vi "LWXPS_OptionalModuleExecute.vi"(6 "LabVIEW error IN":errorcluster, 8 "Module File Name":string, 9 "XPS Reference IN":refnum<k24>) -> (0 "LabVIEW error OUT":errorcluster, 1 "XPS Error String":string, 2 "Returned error code":i32, 3 "XPS Reference OUT":refnum<k24>)   [LabVIEW 2014]
uses:
  D:/XPSQ8_LabView_Library/Development/Source/Dll/Newport.XPS.CommandInterface.dll
  Dll/Newport.XPS.CommandInterface.dll
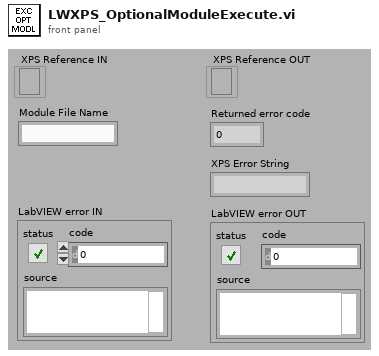
[diagram p1: front panel]
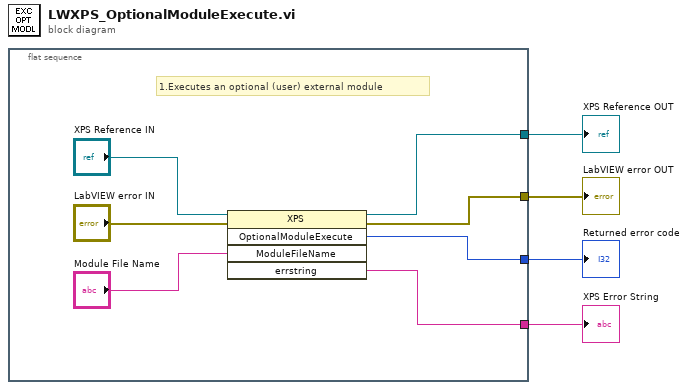
[diagram p0: block diagram]
diagram:
  n1 = flat-sequence {
    tunnel: [w10] -> w4
    tunnel: [w9] -> w3
    tunnel: [w8] -> w2
    tunnel: [w7] -> w1
    frame #0 {
      # "1.Executes an optional (user) external module"
      n2 = invoke class="XPS" method="OptionalModuleExecute"(reference="XPS Reference IN", error in="LabVIEW error IN", "ModuleFileName"="Module File Name") -> (reference out=w9:refnum<k24>, error out=w8:errorcluster, "OptionalModuleExecute"=w7:i32, "errstring"=w10:string)  [unwired: 2 in, 1 out]
    }
  }
  "XPS Error String" <- w4
  "XPS Reference OUT" <- w3
  "LabVIEW error OUT" <- w2
  "Returned error code" <- w1
